vi "Init Queues.vi"(8 "error in (no error)":errorcluster) -> (0 "error out":errorcluster)   [LabVIEW 2016]
uses:
  Controls/Message Structure.ctl
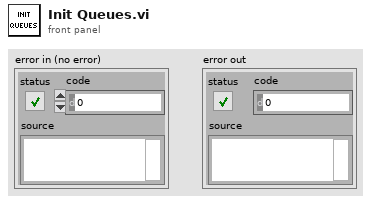
[diagram p1: front panel]
types:
  T1 = typedef "Message Structure.ctl" = cluster{"Data":variant, "Cmd":string}
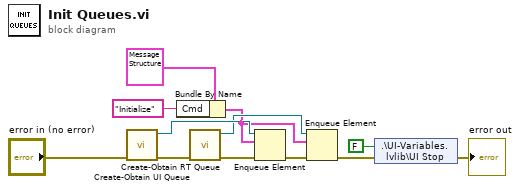
[diagram p0: block diagram]
diagram:
  n1 = call "Create-Obtain UI Queue.vi"("error in (no error)"="error in (no error)") -> ("error out"=w7:errorcluster, "Queue out"=w5:refnum<queue>)  [unwired: 8 in, 1 out]
  n2 = Bundle By Name(cluster=T1 {"Data"=variant, "Cmd"=""} ("Message"), "Cmd"="Initialize") -> (w1:T1)
  n3 = call "Create-Obtain RT Queue.vi"("error in (no error)"=w7) -> ("error out"=w6:errorcluster, "Queue out"=w2:refnum<queue>)  [unwired: 8 in, 1 out]
  n4 = Enqueue Element(queue=w5, element=w1, error in (no error)=w6) -> (error out=w3:errorcluster)  [unwired: 1 in, 2 out]
  n5 = Enqueue Element(queue=w2, element=w1, error in (no error)=w3) -> (error out=w8:errorcluster)  [unwired: 1 in, 2 out]
  n6 = shared-variable ".\\UI-Variables.lvlib\\UI Stop"(FALSE ("UI Stop"), error in=w8) -> (error out=→"error out":errorcluster)
